vi "Init Process.vi"(8 "error in (no error)":errorcluster, 11 "ChartProc in":refnum<class "ChartProc.lvclass">) -> (0 "error out":errorcluster, 3 "ChartProc out":refnum<class "ChartProc.lvclass">)   [LabVIEW 2020, in "LAF2024Q2.lvlib" / "ChartProc.lvclass"]
uses:
  ChartProc.lvclass
  ChartProc.lvclass/ChartProc.ctl
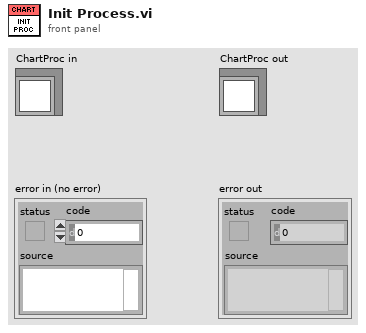
[diagram p1: front panel]
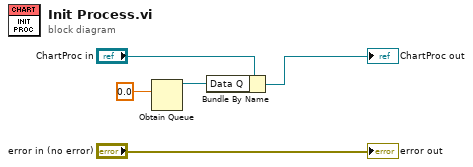
[diagram p0: block diagram]
diagram:
  n1 = Obtain Queue(element data type=0.0) -> (queue out=w1:refnum<queue>)  [unwired: 4 in, 2 out]
  n2 = Bundle By Name(cluster="ChartProc in", "Data Q"=w1) -> (→"ChartProc out":refnum<class "ChartProc.lvclass">)
  "error out" <- "error in (no error)"
